vi "Build Channel Cluster Array.vi"() -> (3 "Channels out":cluster{"Channels":T1[]})   [LabVIEW 2023, in "Cycler Cluster - 24 Channel.lvclass"]
uses:
  Cycler Cluster - 24 Channel.lvclass
  Utilities/Channel.ctl
  Cycler Cluster - 24 Channel.lvclass/Cycler Cluster - 24 Channel.ctl
  Utilities/Utilities.lvlib
panel:
  in  "Cycler Cluster - 24 Channel.lvclass":refnum<class "Cycler Cluster - 24 Channel.lvclass">
  in  "Channels in":cluster{"Channels":T1[]}
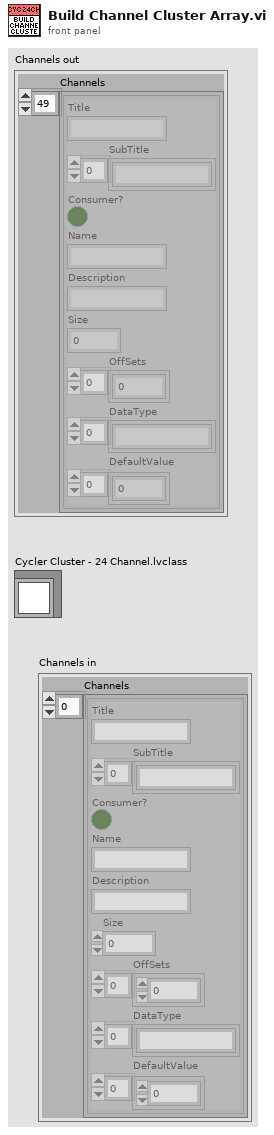
[diagram p1: front panel]
types:
  T1 = typedef "Utilities.lvlib/Channel.ctl" = cluster{"Title":string, "SubTitle":string[], "Consumer?":bool, "Name":string, "Description":string, "Size":i32, "OffSets":i32[], "DataType":string[], "DefaultValue":dbl[]}
  T2 = cluster{"Error.ch01.STS":i32, "OutputEnable.ch01.STS":i32, "ControlMode.ch01.STS":u16, "Voltage.ch01.AV":dbl, "Current.ch01.AV":dbl, "Power.ch01.AV":dbl, "VoltageNominal.ch01.AV":dbl, "CurrentNominal.ch01.AV":dbl, "PowerNominal.ch01.AV":dbl, "ParameterSet.ch01.STS":i32}
  T3 = cluster{"ErrorAcknowledge.ch02.ACT":bool, "OutputEnable.ch02.ACT":bool, "ControlMode.ch02.CTL":u16, "Voltage.ch02.SP":dbl, "VoltageMIN.ch02.SP":dbl, "VoltageMAX.ch02.SP":dbl, "VoltageGrad.ch02.SP":dbl, "Current.ch02.SP":dbl, "CurrentMIN.ch02.SP":dbl, "CurrentMAX.ch02.SP":dbl, "CurrentGrad.ch02.SP":dbl, "Power.ch02.SP":dbl, "PowerMIN.ch02.SP":dbl, "PowerMAX.ch02.SP":dbl, "PowerGrad.ch02.SP":dbl, "ParameterSet.ch02.CTL":i32}
  T4 = cluster{"Error.ch02.STS":i32, "OutputEnable.ch02.STS":i32, "ControlMode.ch02.STS":u16, "Voltage.ch02.AV":dbl, "Current.ch02.AV":dbl, "Power.ch02.AV":dbl, "VoltageNominal.ch02.AV":dbl, "CurrentNominal.ch02.AV":dbl, "PowerNominal.ch02.AV":dbl, "ParameterSet.ch02.STS":i32}
  T5 = cluster{"ErrorAcknowledge.ch03.ACT":bool, "OutputEnable.ch03.ACT":bool, "ControlMode.ch03.CTL":u16, "Voltage.ch03.SP":dbl, "VoltageMIN.ch03.SP":dbl, "VoltageMAX.ch03.SP":dbl, "VoltageGrad.ch03.SP":dbl, "Current.ch03.SP":dbl, "CurrentMIN.ch03.SP":dbl, "CurrentMAX.ch03.SP":dbl, "CurrentGrad.ch03.SP":dbl, "Power.ch03.SP":dbl, "PowerMIN.ch03.SP":dbl, "PowerMAX.ch03.SP":dbl, "PowerGrad.ch03.SP":dbl, "ParameterSet.ch03.CTL":i32}
  T6 = cluster{"Error.ch03.STS":i32, "OutputEnable.ch03.STS":i32, "ControlMode.ch03.STS":u16, "Voltage.ch03.AV":dbl, "Current.ch03.AV":dbl, "Power.ch03.AV":dbl, "VoltageNominal.ch03.AV":dbl, "CurrentNominal.ch03.AV":dbl, "PowerNominal.ch03.AV":dbl, "ParameterSet.ch03.STS":i32}
  T7 = cluster{"ErrorAcknowledge.ch04.ACT":bool, "OutputEnable.ch04.ACT":bool, "ControlMode.ch04.CTL":u16, "Voltage.ch04.SP":dbl, "VoltageMIN.ch04.SP":dbl, "VoltageMAX.ch04.SP":dbl, "VoltageGrad.ch04.SP":dbl, "Current.ch04.SP":dbl, "CurrentMIN.ch04.SP":dbl, "CurrentMAX.ch04.SP":dbl, "CurrentGrad.ch04.SP":dbl, "Power.ch04.SP":dbl, "PowerMIN.ch04.SP":dbl, "PowerMAX.ch04.SP":dbl, "PowerGrad.ch04.SP":dbl, "ParameterSet.ch04.CTL":i32}
  T8 = cluster{"Error.ch04.STS":i32, "OutputEnable.ch04.STS":i32, "ControlMode.ch04.STS":u16, "Voltage.ch04.AV":dbl, "Current.ch04.AV":dbl, "Power.ch04.AV":dbl, "VoltageNominal.ch04.AV":dbl, "CurrentNominal.ch04.AV":dbl, "PowerNominal.ch04.AV":dbl, "ParameterSet.ch04.STS":i32}
  T9 = cluster{"ErrorAcknowledge.ch05.ACT":bool, "OutputEnable.ch05.ACT":bool, "ControlMode.ch05.CTL":u16, "Voltage.ch05.SP":dbl, "VoltageMIN.ch05.SP":dbl, "VoltageMAX.ch05.SP":dbl, "VoltageGrad.ch05.SP":dbl, "Current.ch05.SP":dbl, "CurrentMIN.ch05.SP":dbl, "CurrentMAX.ch05.SP":dbl, "CurrentGrad.ch05.SP":dbl, "Power.ch05.SP":dbl, "PowerMIN.ch05.SP":dbl, "PowerMAX.ch05.SP":dbl, "PowerGrad.ch05.SP":dbl, "ParameterSet.ch05.CTL":i32}
  T10 = cluster{"Error.ch05.STS":i32, "OutputEnable.ch05.STS":i32, "ControlMode.ch05.STS":u16, "Voltage.ch05.AV":dbl, "Current.ch05.AV":dbl, "Power.ch05.AV":dbl, "VoltageNominal.ch05.AV":dbl, "CurrentNominal.ch05.AV":dbl, "PowerNominal.ch05.AV":dbl, "ParameterSet.ch05.STS":i32}
  T11 = cluster{"ErrorAcknowledge.ch06.ACT":bool, "OutputEnable.ch06.ACT":bool, "ControlMode.ch06.CTL":u16, "Voltage.ch06.SP":dbl, "VoltageMIN.ch06.SP":dbl, "VoltageMAX.ch06.SP":dbl, "VoltageGrad.ch06.SP":dbl, "Current.ch06.SP":dbl, "CurrentMIN.ch06.SP":dbl, "CurrentMAX.ch06.SP":dbl, "CurrentGrad.ch06.SP":dbl, "Power.ch06.SP":dbl, "PowerMIN.ch06.SP":dbl, "PowerMAX.ch06.SP":dbl, "PowerGrad.ch06.SP":dbl, "ParameterSet.ch06.CTL":i32}
  T12 = cluster{"Error.ch06.STS":i32, "OutputEnable.ch06.STS":i32, "ControlMode.ch06.STS":u16, "Voltage.ch06.AV":dbl, "Current.ch06.AV":dbl, "Power.ch06.AV":dbl, "VoltageNominal.ch06.AV":dbl, "CurrentNominal.ch06.AV":dbl, "PowerNominal.ch06.AV":dbl, "ParameterSet.ch06.STS":i32}
  T13 = cluster{"ErrorAcknowledge.ch07.ACT":bool, "OutputEnable.ch07.ACT":bool, "ControlMode.ch07.CTL":u16, "Voltage.ch07.SP":dbl, "VoltageMIN.ch07.SP":dbl, "VoltageMAX.ch07.SP":dbl, "VoltageGrad.ch07.SP":dbl, "Current.ch07.SP":dbl, "CurrentMIN.ch07.SP":dbl, "CurrentMAX.ch07.SP":dbl, "CurrentGrad.ch07.SP":dbl, "Power.ch07.SP":dbl, "PowerMIN.ch07.SP":dbl, "PowerMAX.ch07.SP":dbl, "PowerGrad.ch07.SP":dbl, "ParameterSet.ch07.CTL":i32}
  T14 = cluster{"Error.ch07.STS":i32, "OutputEnable.ch07.STS":i32, "ControlMode.ch07.STS":u16, "Voltage.ch07.AV":dbl, "Current.ch07.AV":dbl, "Power.ch07.AV":dbl, "VoltageNominal.ch07.AV":dbl, "CurrentNominal.ch07.AV":dbl, "PowerNominal.ch07.AV":dbl, "ParameterSet.ch07.STS":i32}
  T15 = cluster{"ErrorAcknowledge.ch08.ACT":bool, "OutputEnable.ch08.ACT":bool, "ControlMode.ch08.CTL":u16, "Voltage.ch08.SP":dbl, "VoltageMIN.ch08.SP":dbl, "VoltageMAX.ch08.SP":dbl, "VoltageGrad.ch08.SP":dbl, "Current.ch08.SP":dbl, "CurrentMIN.ch08.SP":dbl, "CurrentMAX.ch08.SP":dbl, "CurrentGrad.ch08.SP":dbl, "Power.ch08.SP":dbl, "PowerMIN.ch08.SP":dbl, "PowerMAX.ch08.SP":dbl, "PowerGrad.ch08.SP":dbl, "ParameterSet.ch08.CTL":i32}
  T16 = cluster{"Error.ch08.STS":i32, "OutputEnable.ch08.STS":i32, "ControlMode.ch08.STS":u16, "Voltage.ch08.AV":dbl, "Current.ch08.AV":dbl, "Power.ch08.AV":dbl, "VoltageNominal.ch08.AV":dbl, "CurrentNominal.ch08.AV":dbl, "PowerNominal.ch08.AV":dbl, "ParameterSet.ch08.STS":i32}
  T17 = cluster{"ErrorAcknowledge.ch09.ACT":bool, "OutputEnable.ch09.ACT":bool, "ControlMode.ch09.CTL":u16, "Voltage.ch09.SP":dbl, "VoltageMIN.ch09.SP":dbl, "VoltageMAX.ch09.SP":dbl, "VoltageGrad.ch09.SP":dbl, "Current.ch09.SP":dbl, "CurrentMIN.ch09.SP":dbl, "CurrentMAX.ch09.SP":dbl, "CurrentGrad.ch09.SP":dbl, "Power.ch09.SP":dbl, "PowerMIN.ch09.SP":dbl, "PowerMAX.ch09.SP":dbl, "PowerGrad.ch09.SP":dbl, "ParameterSet.ch09.CTL":i32}
  T18 = cluster{"Error.ch09.STS":i32, "OutputEnable.ch09.STS":i32, "ControlMode.ch09.STS":u16, "Voltage.ch09.AV":dbl, "Current.ch09.AV":dbl, "Power.ch09.AV":dbl, "VoltageNominal.ch09.AV":dbl, "CurrentNominal.ch09.AV":dbl, "PowerNominal.ch09.AV":dbl, "ParameterSet.ch09.STS":i32}
  T19 = cluster{"ErrorAcknowledge.ch10.ACT":bool, "OutputEnable.ch10.ACT":bool, "ControlMode.ch10.CTL":u16, "Voltage.ch10.SP":dbl, "VoltageMIN.ch10.SP":dbl, "VoltageMAX.ch10.SP":dbl, "VoltageGrad.ch10.SP":dbl, "Current.ch10.SP":dbl, "CurrentMIN.ch10.SP":dbl, "CurrentMAX.ch10.SP":dbl, "CurrentGrad.ch10.SP":dbl, "Power.ch10.SP":dbl, "PowerMIN.ch10.SP":dbl, "PowerMAX.ch10.SP":dbl, "PowerGrad.ch10.SP":dbl, "ParameterSet.ch10.CTL":i32}
  T20 = cluster{"Error.ch10.STS":i32, "OutputEnable.ch10.STS":i32, "ControlMode.ch10.STS":u16, "Voltage.ch10.AV":dbl, "Current.ch10.AV":dbl, "Power.ch10.AV":dbl, "VoltageNominal.ch10.AV":dbl, "CurrentNominal.ch10.AV":dbl, "PowerNominal.ch10.AV":dbl, "ParameterSet.ch10.STS":i32}
  T21 = cluster{"ErrorAcknowledge.ch11.ACT":bool, "OutputEnable.ch11.ACT":bool, "ControlMode.ch11.CTL":u16, "Voltage.ch11.SP":dbl, "VoltageMIN.ch11.SP":dbl, "VoltageMAX.ch11.SP":dbl, "VoltageGrad.ch11.SP":dbl, "Current.ch11.SP":dbl, "CurrentMIN.ch11.SP":dbl, "CurrentMAX.ch11.SP":dbl, "CurrentGrad.ch11.SP":dbl, "Power.ch11.SP":dbl, "PowerMIN.ch11.SP":dbl, "PowerMAX.ch11.SP":dbl, "PowerGrad.ch11.SP":dbl, "ParameterSet.ch11.CTL":i32}
  T22 = cluster{"Error.ch11.STS":i32, "OutputEnable.ch11.STS":i32, "ControlMode.ch11.STS":u16, "Voltage.ch11.AV":dbl, "Current.ch11.AV":dbl, "Power.ch11.AV":dbl, "VoltageNominal.ch11.AV":dbl, "CurrentNominal.ch11.AV":dbl, "PowerNominal.ch11.AV":dbl, "ParameterSet.ch11.STS":i32}
  T23 = cluster{"ErrorAcknowledge.ch12.ACT":bool, "OutputEnable.ch12.ACT":bool, "ControlMode.ch12.CTL":u16, "Voltage.ch12.SP":dbl, "VoltageMIN.ch12.SP":dbl, "VoltageMAX.ch12.SP":dbl, "VoltageGrad.ch12.SP":dbl, "Current.ch12.SP":dbl, "CurrentMIN.ch12.SP":dbl, "CurrentMAX.ch12.SP":dbl, "CurrentGrad.ch12.SP":dbl, "Power.ch12.SP":dbl, "PowerMIN.ch12.SP":dbl, "PowerMAX.ch12.SP":dbl, "PowerGrad.ch12.SP":dbl, "ParameterSet.ch12.CTL":i32}
  T24 = cluster{"Error.ch12.STS":i32, "OutputEnable.ch12.STS":i32, "ControlMode.ch12.STS":u16, "Voltage.ch12.AV":dbl, "Current.ch12.AV":dbl, "Power.ch12.AV":dbl, "VoltageNominal.ch12.AV":dbl, "CurrentNominal.ch12.AV":dbl, "PowerNominal.ch12.AV":dbl, "ParameterSet.ch12.STS":i32}
  T25 = cluster{"ErrorAcknowledge.ch13.ACT":bool, "OutputEnable.ch13.ACT":bool, "ControlMode.ch13.CTL":u16, "Voltage.ch13.SP":dbl, "VoltageMIN.ch13.SP":dbl, "VoltageMAX.ch13.SP":dbl, "VoltageGrad.ch13.SP":dbl, "Current.ch13.SP":dbl, "CurrentMIN.ch13.SP":dbl, "CurrentMAX.ch13.SP":dbl, "CurrentGrad.ch13.SP":dbl, "Power.ch13.SP":dbl, "PowerMIN.ch13.SP":dbl, "PowerMAX.ch13.SP":dbl, "PowerGrad.ch13.SP":dbl, "ParameterSet.ch13.CTL":i32}
  T26 = cluster{"Error.ch13.STS":i32, "OutputEnable.ch13.STS":i32, "ControlMode.ch13.STS":u16, "Voltage.ch13.AV":dbl, "Current.ch13.AV":dbl, "Power.ch13.AV":dbl, "VoltageNominal.ch13.AV":dbl, "CurrentNominal.ch13.AV":dbl, "PowerNominal.ch13.AV":dbl, "ParameterSet.ch13.STS":i32}
  T27 = cluster{"ErrorAcknowledge.ch14.ACT":bool, "OutputEnable.ch14.ACT":bool, "ControlMode.ch14.CTL":u16, "Voltage.ch14.SP":dbl, "VoltageMIN.ch14.SP":dbl, "VoltageMAX.ch14.SP":dbl, "VoltageGrad.ch14.SP":dbl, "Current.ch14.SP":dbl, "CurrentMIN.ch14.SP":dbl, "CurrentMAX.ch14.SP":dbl, "CurrentGrad.ch14.SP":dbl, "Power.ch14.SP":dbl, "PowerMIN.ch14.SP":dbl, "PowerMAX.ch14.SP":dbl, "PowerGrad.ch14.SP":dbl, "ParameterSet.ch14.CTL":i32}
  T28 = cluster{"Error.ch14.STS":i32, "OutputEnable.ch14.STS":i32, "ControlMode.ch14.STS":u16, "Voltage.ch14.AV":dbl, "Current.ch14.AV":dbl, "Power.ch14.AV":dbl, "VoltageNominal.ch14.AV":dbl, "CurrentNominal.ch14.AV":dbl, "PowerNominal.ch14.AV":dbl, "ParameterSet.ch14.STS":i32}
  T29 = cluster{"ErrorAcknowledge.ch15.ACT":bool, "OutputEnable.ch15.ACT":bool, "ControlMode.ch15.CTL":u16, "Voltage.ch15.SP":dbl, "VoltageMIN.ch15.SP":dbl, "VoltageMAX.ch15.SP":dbl, "VoltageGrad.ch15.SP":dbl, "Current.ch15.SP":dbl, "CurrentMIN.ch15.SP":dbl, "CurrentMAX.ch15.SP":dbl, "CurrentGrad.ch15.SP":dbl, "Power.ch15.SP":dbl, "PowerMIN.ch15.SP":dbl, "PowerMAX.ch15.SP":dbl, "PowerGrad.ch15.SP":dbl, "ParameterSet.ch15.CTL":i32}
  T30 = cluster{"Error.ch15.STS":i32, "OutputEnable.ch15.STS":i32, "ControlMode.ch15.STS":u16, "Voltage.ch15.AV":dbl, "Current.ch15.AV":dbl, "Power.ch15.AV":dbl, "VoltageNominal.ch15.AV":dbl, "CurrentNominal.ch15.AV":dbl, "PowerNominal.ch15.AV":dbl, "ParameterSet.ch15.STS":i32}
  T31 = cluster{"ErrorAcknowledge.ch16.ACT":bool, "OutputEnable.ch16.ACT":bool, "ControlMode.ch16.CTL":u16, "Voltage.ch16.SP":dbl, "VoltageMIN.ch16.SP":dbl, "VoltageMAX.ch16.SP":dbl, "VoltageGrad.ch16.SP":dbl, "Current.ch16.SP":dbl, "CurrentMIN.ch16.SP":dbl, "CurrentMAX.ch16.SP":dbl, "CurrentGrad.ch16.SP":dbl, "Power.ch16.SP":dbl, "PowerMIN.ch16.SP":dbl, "PowerMAX.ch16.SP":dbl, "PowerGrad.ch16.SP":dbl, "ParameterSet.ch16.CTL":i32}
  T32 = cluster{"Error.ch16.STS":i32, "OutputEnable.ch16.STS":i32, "ControlMode.ch16.STS":u16, "Voltage.ch16.AV":dbl, "Current.ch16.AV":dbl, "Power.ch16.AV":dbl, "VoltageNominal.ch16.AV":dbl, "CurrentNominal.ch16.AV":dbl, "PowerNominal.ch16.AV":dbl, "ParameterSet.ch16.STS":i32}
  T33 = cluster{"ErrorAcknowledge.ch17.ACT":bool, "OutputEnable.ch17.ACT":bool, "ControlMode.ch17.CTL":u16, "Voltage.ch17.SP":dbl, "VoltageMIN.ch17.SP":dbl, "VoltageMAX.ch17.SP":dbl, "VoltageGrad.ch17.SP":dbl, "Current.ch17.SP":dbl, "CurrentMIN.ch17.SP":dbl, "CurrentMAX.ch17.SP":dbl, "CurrentGrad.ch17.SP":dbl, "Power.ch17.SP":dbl, "PowerMIN.ch17.SP":dbl, "PowerMAX.ch17.SP":dbl, "PowerGrad.ch17.SP":dbl, "ParameterSet.ch17.CTL":i32}
  T34 = cluster{"Error.ch17.STS":i32, "OutputEnable.ch17.STS":i32, "ControlMode.ch17.STS":u16, "Voltage.ch17.AV":dbl, "Current.ch17.AV":dbl, "Power.ch17.AV":dbl, "VoltageNominal.ch17.AV":dbl, "CurrentNominal.ch17.AV":dbl, "PowerNominal.ch17.AV":dbl, "ParameterSet.ch17.STS":i32}
  T35 = cluster{"ErrorAcknowledge.ch18.ACT":bool, "OutputEnable.ch18.ACT":bool, "ControlMode.ch18.CTL":u16, "Voltage.ch18.SP":dbl, "VoltageMIN.ch18.SP":dbl, "VoltageMAX.ch18.SP":dbl, "VoltageGrad.ch18.SP":dbl, "Current.ch18.SP":dbl, "CurrentMIN.ch18.SP":dbl, "CurrentMAX.ch18.SP":dbl, "CurrentGrad.ch18.SP":dbl, "Power.ch18.SP":dbl, "PowerMIN.ch18.SP":dbl, "PowerMAX.ch18.SP":dbl, "PowerGrad.ch18.SP":dbl, "ParameterSet.ch18.CTL":i32}
  T36 = cluster{"Error.ch18.STS":i32, "OutputEnable.ch18.STS":i32, "ControlMode.ch18.STS":u16, "Voltage.ch18.AV":dbl, "Current.ch18.AV":dbl, "Power.ch18.AV":dbl, "VoltageNominal.ch18.AV":dbl, "CurrentNominal.ch18.AV":dbl, "PowerNominal.ch18.AV":dbl, "ParameterSet.ch18.STS":i32}
  T37 = cluster{"ErrorAcknowledge.ch19.ACT":bool, "OutputEnable.ch19.ACT":bool, "ControlMode.ch19.CTL":u16, "Voltage.ch19.SP":dbl, "VoltageMIN.ch19.SP":dbl, "VoltageMAX.ch19.SP":dbl, "VoltageGrad.ch19.SP":dbl, "Current.ch19.SP":dbl, "CurrentMIN.ch19.SP":dbl, "CurrentMAX.ch19.SP":dbl, "CurrentGrad.ch19.SP":dbl, "Power.ch19.SP":dbl, "PowerMIN.ch19.SP":dbl, "PowerMAX.ch19.SP":dbl, "PowerGrad.ch19.SP":dbl, "ParameterSet.ch19.CTL":i32}
  T38 = cluster{"Error.ch19.STS":i32, "OutputEnable.ch19.STS":i32, "ControlMode.ch19.STS":u16, "Voltage.ch19.AV":dbl, "Current.ch19.AV":dbl, "Power.ch19.AV":dbl, "VoltageNominal.ch19.AV":dbl, "CurrentNominal.ch19.AV":dbl, "PowerNominal.ch19.AV":dbl, "ParameterSet.ch19.STS":i32}
  T39 = cluster{"ErrorAcknowledge.ch20.ACT":bool, "OutputEnable.ch20.ACT":bool, "ControlMode.ch20.CTL":u16, "Voltage.ch20.SP":dbl, "VoltageMIN.ch20.SP":dbl, "VoltageMAX.ch20.SP":dbl, "VoltageGrad.ch20.SP":dbl, "Current.ch20.SP":dbl, "CurrentMIN.ch20.SP":dbl, "CurrentMAX.ch20.SP":dbl, "CurrentGrad.ch20.SP":dbl, "Power.ch20.SP":dbl, "PowerMIN.ch20.SP":dbl, "PowerMAX.ch20.SP":dbl, "PowerGrad.ch20.SP":dbl, "ParameterSet.ch20.CTL":i32}
  T40 = cluster{"Error.ch20.STS":i32, "OutputEnable.ch20.STS":i32, "ControlMode.ch20.STS":u16, "Voltage.ch20.AV":dbl, "Current.ch20.AV":dbl, "Power.ch20.AV":dbl, "VoltageNominal.ch20.AV":dbl, "CurrentNominal.ch20.AV":dbl, "PowerNominal.ch20.AV":dbl, "ParameterSet.ch20.STS":i32}
  T41 = cluster{"ErrorAcknowledge.ch21.ACT":bool, "OutputEnable.ch21.ACT":bool, "ControlMode.ch21.CTL":u16, "Voltage.ch21.SP":dbl, "VoltageMIN.ch21.SP":dbl, "VoltageMAX.ch21.SP":dbl, "VoltageGrad.ch21.SP":dbl, "Current.ch21.SP":dbl, "CurrentMIN.ch21.SP":dbl, "CurrentMAX.ch21.SP":dbl, "CurrentGrad.ch21.SP":dbl, "Power.ch21.SP":dbl, "PowerMIN.ch21.SP":dbl, "PowerMAX.ch21.SP":dbl, "PowerGrad.ch21.SP":dbl, "ParameterSet.ch21.CTL":i32}
  T42 = cluster{"Error.ch21.STS":i32, "OutputEnable.ch21.STS":i32, "ControlMode.ch21.STS":u16, "Voltage.ch21.AV":dbl, "Current.ch21.AV":dbl, "Power.ch21.AV":dbl, "VoltageNominal.ch21.AV":dbl, "CurrentNominal.ch21.AV":dbl, "PowerNominal.ch21.AV":dbl, "ParameterSet.ch21.STS":i32}
  T43 = cluster{"ErrorAcknowledge.ch22.ACT":bool, "OutputEnable.ch22.ACT":bool, "ControlMode.ch22.CTL":u16, "Voltage.ch22.SP":dbl, "VoltageMIN.ch22.SP":dbl, "VoltageMAX.ch22.SP":dbl, "VoltageGrad.ch22.SP":dbl, "Current.ch22.SP":dbl, "CurrentMIN.ch22.SP":dbl, "CurrentMAX.ch22.SP":dbl, "CurrentGrad.ch22.SP":dbl, "Power.ch22.SP":dbl, "PowerMIN.ch22.SP":dbl, "PowerMAX.ch22.SP":dbl, "PowerGrad.ch22.SP":dbl, "ParameterSet.ch22.CTL":i32}
  T44 = cluster{"Error.ch22.STS":i32, "OutputEnable.ch22.STS":i32, "ControlMode.ch22.STS":u16, "Voltage.ch22.AV":dbl, "Current.ch22.AV":dbl, "Power.ch22.AV":dbl, "VoltageNominal.ch22.AV":dbl, "CurrentNominal.ch22.AV":dbl, "PowerNominal.ch22.AV":dbl, "ParameterSet.ch22.STS":i32}
  T45 = cluster{"ErrorAcknowledge.ch23.ACT":bool, "OutputEnable.ch23.ACT":bool, "ControlMode.ch23.CTL":u16, "Voltage.ch23.SP":dbl, "VoltageMIN.ch23.SP":dbl, "VoltageMAX.ch23.SP":dbl, "VoltageGrad.ch23.SP":dbl, "Current.ch23.SP":dbl, "CurrentMIN.ch23.SP":dbl, "CurrentMAX.ch23.SP":dbl, "CurrentGrad.ch23.SP":dbl, "Power.ch23.SP":dbl, "PowerMIN.ch23.SP":dbl, "PowerMAX.ch23.SP":dbl, "PowerGrad.ch23.SP":dbl, "ParameterSet.ch23.CTL":i32}
  T46 = cluster{"Error.ch23.STS":i32, "OutputEnable.ch23.STS":i32, "ControlMode.ch23.STS":u16, "Voltage.ch23.AV":dbl, "Current.ch23.AV":dbl, "Power.ch23.AV":dbl, "VoltageNominal.ch23.AV":dbl, "CurrentNominal.ch23.AV":dbl, "PowerNominal.ch23.AV":dbl, "ParameterSet.ch23.STS":i32}
  T47 = cluster{"ErrorAcknowledge.ch24.ACT":bool, "OutputEnable.ch24.ACT":bool, "ControlMode.ch24.CTL":u16, "Voltage.ch24.SP":dbl, "VoltageMIN.ch24.SP":dbl, "VoltageMAX.ch24.SP":dbl, "VoltageGrad.ch24.SP":dbl, "Current.ch24.SP":dbl, "CurrentMIN.ch24.SP":dbl, "CurrentMAX.ch24.SP":dbl, "CurrentGrad.ch24.SP":dbl, "Power.ch24.SP":dbl, "PowerMIN.ch24.SP":dbl, "PowerMAX.ch24.SP":dbl, "PowerGrad.ch24.SP":dbl, "ParameterSet.ch24.CTL":i32}
  T48 = cluster{"Error.ch24.STS":i32, "OutputEnable.ch24.STS":i32, "ControlMode.ch24.STS":u16, "Voltage.ch24.AV":dbl, "Current.ch24.AV":dbl, "Power.ch24.AV":dbl, "VoltageNominal.ch24.AV":dbl, "CurrentNominal.ch24.AV":dbl, "PowerNominal.ch24.AV":dbl, "ParameterSet.ch24.STS":i32}
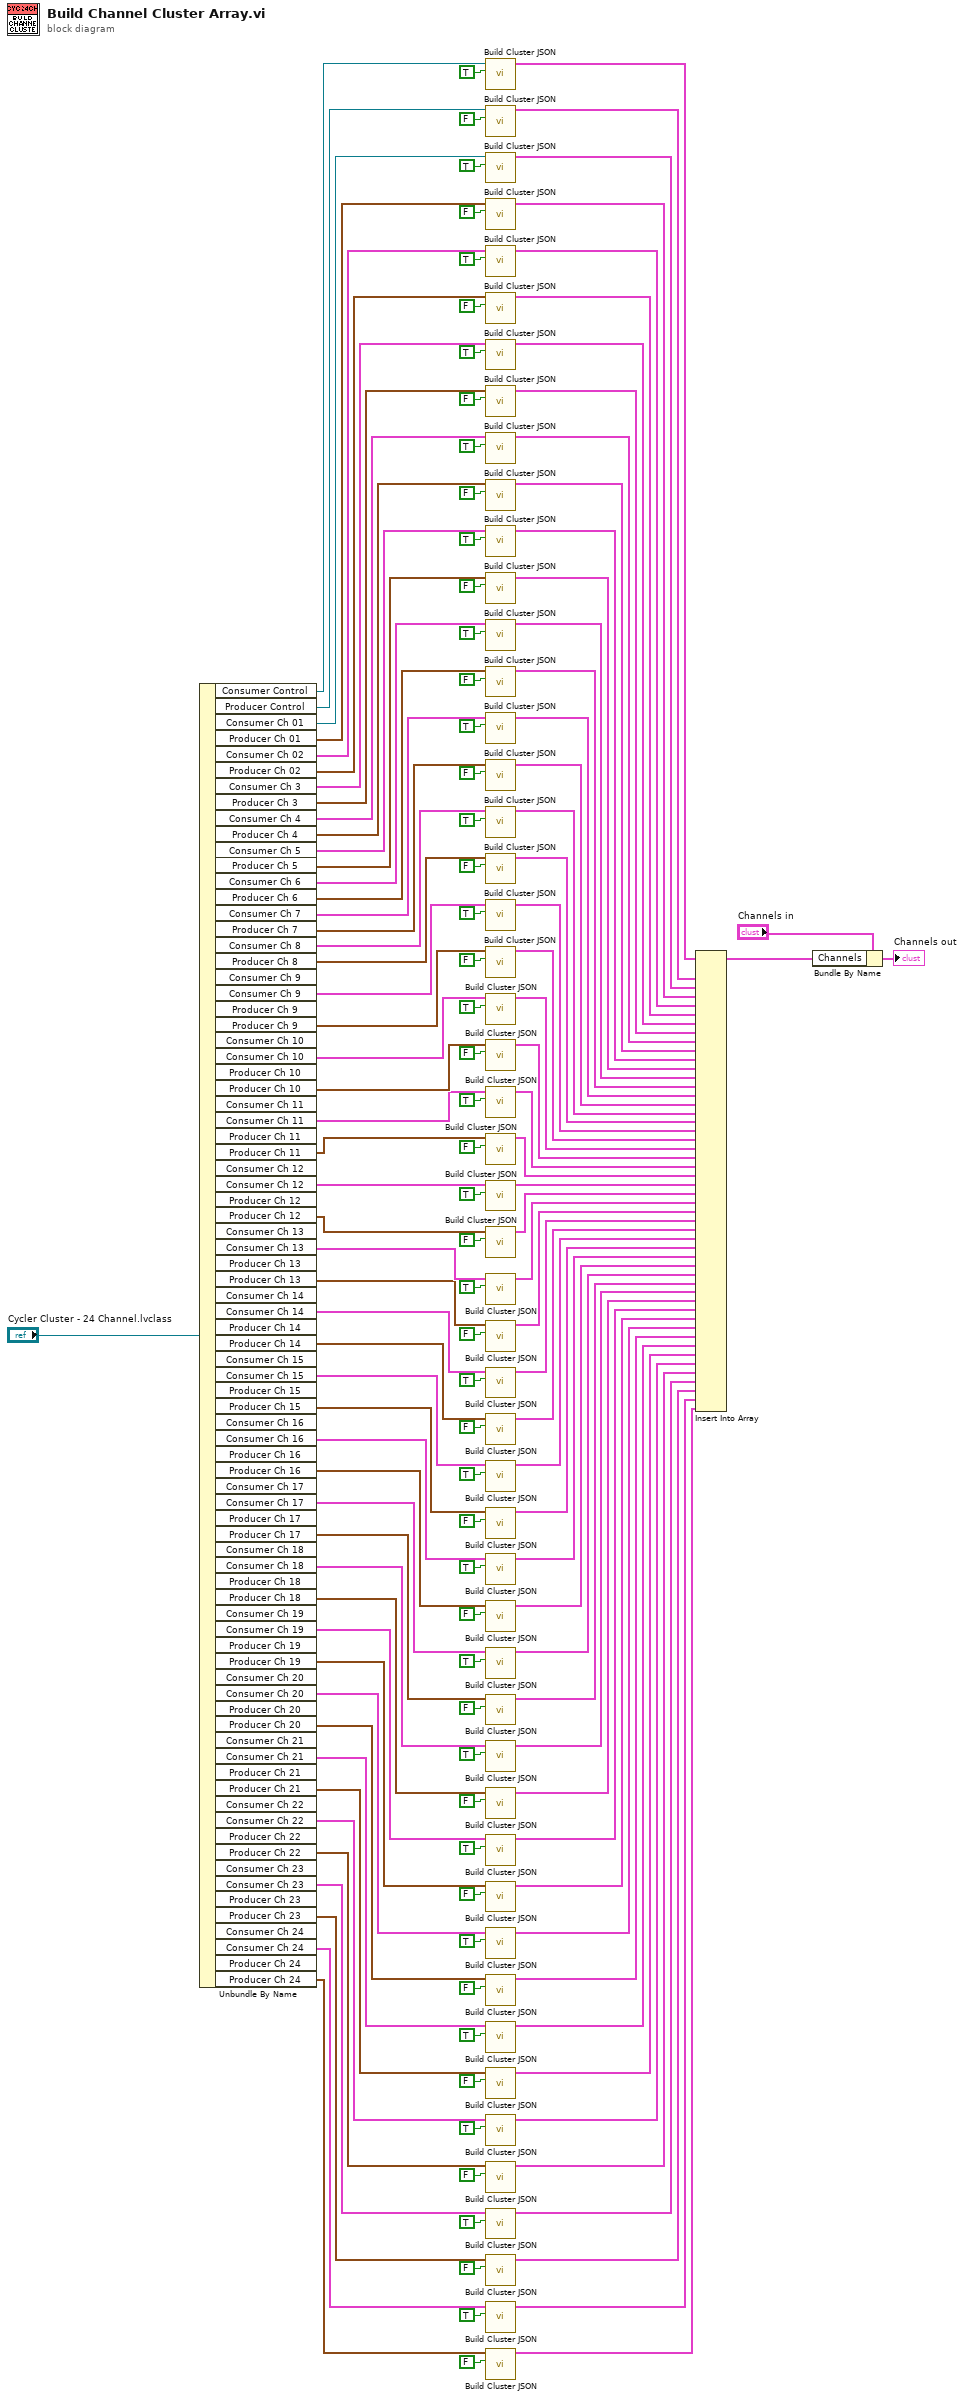
[diagram p0: block diagram]
diagram:
  n1 = Unbundle By Name("Cycler Cluster - 24 Channel.lvclass") -> ("Consumer Control"=w154:refnum<k21>, "Producer Control"=w153:refnum<k21>, "Consumer Ch 01"=w142:refnum<k21>, "Producer Ch 01"=w143:T2, "Consumer Ch 02"=w135:T3, "Producer Ch 02"=w134:T4, "Consumer Ch 3"=w91:T5, "Producer Ch 3"=w90:T6, "Consumer Ch 4"=w89:T7, "Producer Ch 4"=w88:T8, "Consumer Ch 5"=w87:T9, "Producer Ch 5"=w86:T10, "Consumer Ch 6"=w85:T11, "Producer Ch 6"=w84:T12, "Consumer Ch 7"=w83:T13, "Producer Ch 7"=w82:T14, "Consumer Ch 8"=w81:T15, "Producer Ch 8"=w80:T16, "Consumer Ch 9"=w79:T17, "Producer Ch 9"=w78:T18, "Consumer Ch 10"=w77:T19, "Producer Ch 10"=w76:T20, "Consumer Ch 11"=w75:T21, "Producer Ch 11"=w74:T22, "Consumer Ch 12"=w73:T23, "Producer Ch 12"=w72:T24, "Consumer Ch 13"=w71:T25, "Producer Ch 13"=w70:T26, "Consumer Ch 14"=w69:T27, "Producer Ch 14"=w67:T28, "Consumer Ch 15"=w66:T29, "Producer Ch 15"=w65:T30, "Consumer Ch 16"=w64:T31, "Producer Ch 16"=w63:T32, "Consumer Ch 17"=w62:T33, "Producer Ch 17"=w61:T34, "Consumer Ch 18"=w60:T35, "Producer Ch 18"=w59:T36, "Consumer Ch 19"=w58:T37, "Producer Ch 19"=w57:T38, "Consumer Ch 20"=w55:T39, "Producer Ch 20"=w53:T40, "Consumer Ch 21"=w54:T41, "Producer Ch 21"=w51:T42, "Consumer Ch 22"=w50:T43, "Producer Ch 22"=w49:T44, "Consumer Ch 23"=w48:T45, "Producer Ch 23"=w47:T46, "Consumer Ch 24"=w46:T47, "Producer Ch 24"=w45:T48)  [unwired: 32 out]
  n2 = call "Build Cluster JSON.vi"("Consumer?"=TRUE, "Cluster"=w154) -> ("Array"=w150:T1[])  [unwired: 9 in]
  n3 = call "Build Cluster JSON.vi"("Consumer?"=FALSE, "Cluster"=w153) -> ("Array"=w149:T1[])  [unwired: 9 in]
  n4 = call "Build Cluster JSON.vi"("Consumer?"=TRUE, "Cluster"=w142) -> ("Array"=w141:T1[])  [unwired: 9 in]
  n5 = call "Build Cluster JSON.vi"("Consumer?"=FALSE, "Cluster"=w143) -> ("Array"=w140:T1[])  [unwired: 9 in]
  n6 = call "Build Cluster JSON.vi"("Consumer?"=TRUE, "Cluster"=w135) -> ("Array"=w137:T1[])  [unwired: 9 in]
  n7 = call "Build Cluster JSON.vi"("Consumer?"=FALSE, "Cluster"=w134) -> ("Array"=w136:T1[])  [unwired: 9 in]
  n8 = call "Build Cluster JSON.vi"("Consumer?"=TRUE, "Cluster"=w91) -> ("Array"=w44:T1[])  [unwired: 9 in]
  n9 = call "Build Cluster JSON.vi"("Consumer?"=FALSE, "Cluster"=w90) -> ("Array"=w43:T1[])  [unwired: 9 in]
  n10 = call "Build Cluster JSON.vi"("Consumer?"=TRUE, "Cluster"=w89) -> ("Array"=w42:T1[])  [unwired: 9 in]
  n11 = call "Build Cluster JSON.vi"("Consumer?"=FALSE, "Cluster"=w88) -> ("Array"=w41:T1[])  [unwired: 9 in]
  n12 = call "Build Cluster JSON.vi"("Consumer?"=TRUE, "Cluster"=w87) -> ("Array"=w40:T1[])  [unwired: 9 in]
  n13 = call "Build Cluster JSON.vi"("Consumer?"=FALSE, "Cluster"=w86) -> ("Array"=w39:T1[])  [unwired: 9 in]
  n14 = call "Build Cluster JSON.vi"("Consumer?"=TRUE, "Cluster"=w85) -> ("Array"=w38:T1[])  [unwired: 9 in]
  n15 = call "Build Cluster JSON.vi"("Consumer?"=FALSE, "Cluster"=w84) -> ("Array"=w37:T1[])  [unwired: 9 in]
  n16 = call "Build Cluster JSON.vi"("Consumer?"=TRUE, "Cluster"=w83) -> ("Array"=w36:T1[])  [unwired: 9 in]
  n17 = call "Build Cluster JSON.vi"("Consumer?"=FALSE, "Cluster"=w82) -> ("Array"=w35:T1[])  [unwired: 9 in]
  n18 = call "Build Cluster JSON.vi"("Consumer?"=TRUE, "Cluster"=w81) -> ("Array"=w34:T1[])  [unwired: 9 in]
  n19 = call "Build Cluster JSON.vi"("Consumer?"=FALSE, "Cluster"=w80) -> ("Array"=w33:T1[])  [unwired: 9 in]
  n20 = call "Build Cluster JSON.vi"("Consumer?"=TRUE, "Cluster"=w79) -> ("Array"=w32:T1[])  [unwired: 9 in]
  n21 = call "Build Cluster JSON.vi"("Consumer?"=FALSE, "Cluster"=w78) -> ("Array"=w31:T1[])  [unwired: 9 in]
  n22 = call "Build Cluster JSON.vi"("Consumer?"=TRUE, "Cluster"=w77) -> ("Array"=w30:T1[])  [unwired: 9 in]
  n23 = call "Build Cluster JSON.vi"("Consumer?"=FALSE, "Cluster"=w76) -> ("Array"=w29:T1[])  [unwired: 9 in]
  n24 = call "Build Cluster JSON.vi"("Consumer?"=TRUE, "Cluster"=w75) -> ("Array"=w28:T1[])  [unwired: 9 in]
  n25 = call "Build Cluster JSON.vi"("Consumer?"=FALSE, "Cluster"=w74) -> ("Array"=w27:T1[])  [unwired: 9 in]
  n26 = call "Build Cluster JSON.vi"("Consumer?"=TRUE, "Cluster"=w73) -> ("Array"=w26:T1[])  [unwired: 9 in]
  n27 = call "Build Cluster JSON.vi"("Consumer?"=FALSE, "Cluster"=w72) -> ("Array"=w25:T1[])  [unwired: 9 in]
  n28 = call "Build Cluster JSON.vi"("Consumer?"=TRUE, "Cluster"=w71) -> ("Array"=w24:T1[])  [unwired: 9 in]
  n29 = call "Build Cluster JSON.vi"("Consumer?"=FALSE, "Cluster"=w70) -> ("Array"=w23:T1[])  [unwired: 9 in]
  n30 = call "Build Cluster JSON.vi"("Consumer?"=TRUE, "Cluster"=w69) -> ("Array"=w22:T1[])  [unwired: 9 in]
  n31 = call "Build Cluster JSON.vi"("Consumer?"=FALSE, "Cluster"=w67) -> ("Array"=w21:T1[])  [unwired: 9 in]
  n32 = call "Build Cluster JSON.vi"("Consumer?"=TRUE, "Cluster"=w66) -> ("Array"=w20:T1[])  [unwired: 9 in]
  n33 = call "Build Cluster JSON.vi"("Consumer?"=FALSE, "Cluster"=w65) -> ("Array"=w19:T1[])  [unwired: 9 in]
  n34 = call "Build Cluster JSON.vi"("Consumer?"=TRUE, "Cluster"=w64) -> ("Array"=w18:T1[])  [unwired: 9 in]
  n35 = call "Build Cluster JSON.vi"("Consumer?"=FALSE, "Cluster"=w63) -> ("Array"=w17:T1[])  [unwired: 9 in]
  n36 = call "Build Cluster JSON.vi"("Consumer?"=TRUE, "Cluster"=w62) -> ("Array"=w16:T1[])  [unwired: 9 in]
  n37 = call "Build Cluster JSON.vi"("Consumer?"=FALSE, "Cluster"=w61) -> ("Array"=w15:T1[])  [unwired: 9 in]
  n38 = call "Build Cluster JSON.vi"("Consumer?"=TRUE, "Cluster"=w60) -> ("Array"=w14:T1[])  [unwired: 9 in]
  n39 = call "Build Cluster JSON.vi"("Consumer?"=FALSE, "Cluster"=w59) -> ("Array"=w13:T1[])  [unwired: 9 in]
  n40 = call "Build Cluster JSON.vi"("Consumer?"=TRUE, "Cluster"=w58) -> ("Array"=w12:T1[])  [unwired: 9 in]
  n41 = call "Build Cluster JSON.vi"("Consumer?"=FALSE, "Cluster"=w57) -> ("Array"=w11:T1[])  [unwired: 9 in]
  n42 = call "Build Cluster JSON.vi"("Consumer?"=TRUE, "Cluster"=w55) -> ("Array"=w10:T1[])  [unwired: 9 in]
  n43 = call "Build Cluster JSON.vi"("Consumer?"=FALSE, "Cluster"=w53) -> ("Array"=w9:T1[])  [unwired: 9 in]
  n44 = call "Build Cluster JSON.vi"("Consumer?"=TRUE, "Cluster"=w54) -> ("Array"=w8:T1[])  [unwired: 9 in]
  n45 = call "Build Cluster JSON.vi"("Consumer?"=FALSE, "Cluster"=w51) -> ("Array"=w7:T1[])  [unwired: 9 in]
  n46 = call "Build Cluster JSON.vi"("Consumer?"=TRUE, "Cluster"=w50) -> ("Array"=w6:T1[])  [unwired: 9 in]
  n47 = call "Build Cluster JSON.vi"("Consumer?"=FALSE, "Cluster"=w49) -> ("Array"=w5:T1[])  [unwired: 9 in]
  n48 = call "Build Cluster JSON.vi"("Consumer?"=TRUE, "Cluster"=w48) -> ("Array"=w4:T1[])  [unwired: 9 in]
  n49 = call "Build Cluster JSON.vi"("Consumer?"=FALSE, "Cluster"=w47) -> ("Array"=w3:T1[])  [unwired: 9 in]
  n50 = call "Build Cluster JSON.vi"("Consumer?"=TRUE, "Cluster"=w46) -> ("Array"=w2:T1[])  [unwired: 9 in]
  n51 = call "Build Cluster JSON.vi"("Consumer?"=FALSE, "Cluster"=w45) -> ("Array"=w1:T1[])  [unwired: 9 in]
  n52 = Insert Into Array(array=w150, new element #1=w149, new element #2=w141, new element #3=w140, new element #4=w137, new element #5=w136, new element #6=w44, new element #7=w43, new element #8=w42, new element #9=w41, new element #10=w40, new element #11=w39, new element #12=w38, new element #13=w37, new element #14=w36, new element #15=w35, new element #16=w34, new element #17=w33, new element #18=w32, new element #19=w31, new element #20=w30, new element #21=w29, new element #22=w28, new element #23=w27, new element #24=w26, new element #25=w25, new element #26=w24, new element #27=w23, new element #28=w22, new element #29=w21, new element #30=w20, new element #31=w19, new element #32=w18, new element #33=w17, new element #34=w16, new element #35=w15, new element #36=w14, new element #37=w13, new element #38=w12, new element #39=w11, new element #40=w10, new element #41=w9, new element #42=w8, new element #43=w7, new element #44=w6, new element #45=w5, new element #46=w4, new element #47=w3, new element #48=w2, new element #49=w1) -> (w147:T1[])  [unwired: 1 in]
  n53 = Bundle By Name(cluster="Channels in", "Channels"=w147) -> (→"Channels out":cluster{"Channels":T1[]})
